vi "Bounds_origin.vi"(7 "Origin":T2, 11 "Bounds In":T1) -> (3 "Bounds out":T1)   [LabVIEW 2015]
uses:
  <vilib>/Utility/miscctls.llb/LVRectTypeDef.ctl
  <vilib>/Utility/miscctls.llb/LVPointTypeDef.ctl
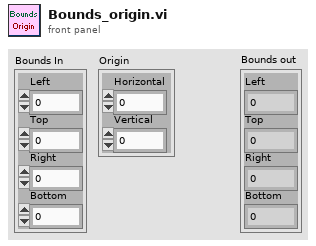
[diagram p1: front panel]
types:
  T1 = typedef "LVRectTypeDef.ctl" = cluster{"Left":i16, "Top":i16, "Right":i16, "Bottom":i16}
  T2 = typedef "LVPointTypeDef.ctl" = cluster{"Horizontal":i16, "Vertical":i16}
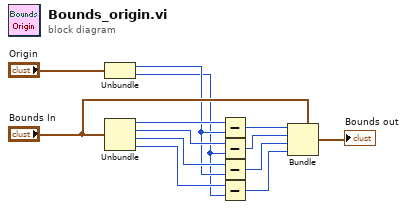
[diagram p0: block diagram]
diagram:
  n1 = Unbundle("Origin") -> ("Horizontal"=w2:i16, "Vertical"=w1:i16)
  n2 = Unbundle("Bounds In") -> ("Left"=w6:i16, "Top"=w5:i16, "Right"=w4:i16, "Bottom"=w3:i16)
  n3 = Subtract(x=w6, y=w2) -> (x-y=w12:i16)
  n4 = Subtract(x=w5, y=w1) -> (x-y=w10:i16)
  n5 = Subtract(x=w4, y=w2) -> (x-y=w9:i16)
  n6 = Subtract(x=w3, y=w1) -> (x-y=w8:i16)
  n7 = Bundle(cluster="Bounds In", "Left"=w12, "Top"=w10, "Right"=w9, "Bottom"=w8) -> (→"Bounds out":T1)
